vi "image_message_to_gemini_message.vi"(2 "error in (no error)":errorcluster, 3 "message":T2) -> (0 "error out":errorcluster, 1 "Content (JSON)":string)   [LabVIEW 2020, in "llm_gemini_chatmodels.lvclass"]
uses:
  llm_gemini_chatmodels.lvclass
  message_image/message.ctl
  message_image/message_image.lvclass
panel:
  out "content":T1
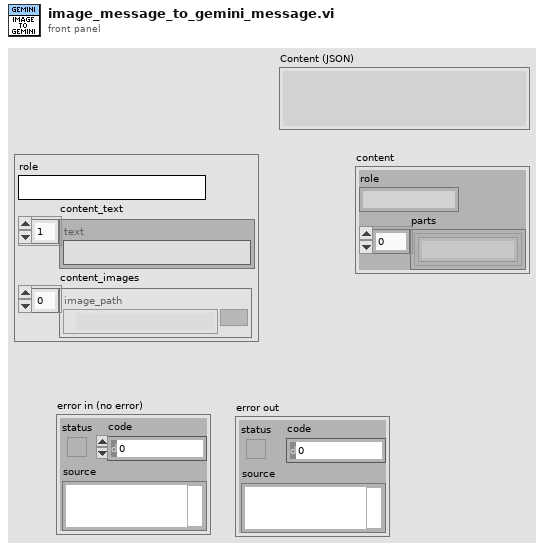
[diagram p1: front panel]
types:
  T1 = cluster{"role":string, "parts":cluster{string}[]}
  T2 = typedef "message_image.lvclass/message.ctl" = cluster{"role":string, "content_text":string[], "content_images":path[]}
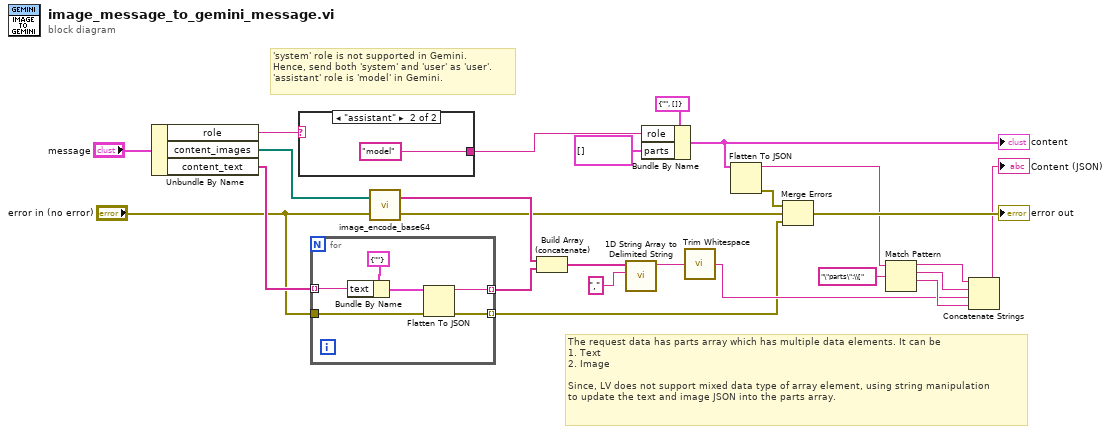
[diagram p0: block diagram]
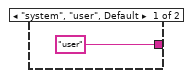
[diagram p2: hidden frame]
diagram:
  # "The request data has parts array which has multiple data elements. It can be \n1. Text\n2. Image\n\nSince, LV does not support mixed data type of array element, using string manipulation\nto update the text and image JSON into the parts array."
  # "'system' role is not supported in Gemini.\nHence, send both 'system' and 'user' as 'user'.\n'assistant' role is 'model' in Gemini."
  n1 = Unbundle By Name("message") -> ("role"=w24:string, "content_images"=w22:path[], "content_text"=w5:string[])
  n2 = case shown="\"assistant\"" w24 {
    tunnel: ["user" ("role") "model" ("role")] -> w23
    frame "system", "user", Default {
    }
    frame "assistant" {
    }
  }
  n3 = for {
    tunnel: w5 -> [w33] mode=indexing
    tunnel: [w30] -> w16 mode=indexing
    tunnel: "error in (no error)" -> [w29]
    tunnel: [w28] -> w4 mode=indexing
    n4 = Bundle By Name(cluster=cluster{"text":string} {"text"=""} ("parts"), "text"=w33) -> (w31:cluster{"text":string})
    n5 = Flatten To JSON(anything=w31, error in (no error)=w29) -> (JSON string=w30:string, 11:w28:errorcluster)  [unwired: 1 in]
  }
  n6 = call "image_encode_base64.vi"("error in (no error)"="error in (no error)", "imagepaths"=w22) -> ("error out"=w3:errorcluster, "image_data"=w17:string[])
  n7 = Build Array (concatenate)(w17, w16) -> (w13:string[])
  n8 = call <vilib>:"1D String Array to Delimited String.vi"("delimiter"=",", "string array"=w13) -> ("delimited string"=w14:string)  [unwired: 9 in]
  n9 = Bundle By Name(cluster=T1 {"role"="", "parts"=[]} ("content"), "role"=w23, "parts"=cluster{string}[] []) -> (w18:T1)
  "content" <- w18
  n10 = call <vilib>:"Trim Whitespace.vi"("string"=w14) -> ("trimmed string"=w8:string)  [unwired: 1 in]
  n11 = Flatten To JSON(anything=w18) -> (JSON string=w7:string, 11:w2:errorcluster)  [unwired: 2 in]
  n12 = Merge Errors(w2, w3, w4) -> (→"error out":errorcluster)
  n13 = Match Pattern(string=w7, regular expression="\"parts\":\\[") -> (before substring=w11:string, match substring=w10:string, after substring=w9:string)  [unwired: 1 in, 1 out]
  n14 = Concatenate Strings(w11, w10, w8, w9) -> (→"Content (JSON)":string)
